vi "hex_ascii.vi"(11 "IN （HEX）":string) -> (3 "ASCII":string)   [LabVIEW 2015]
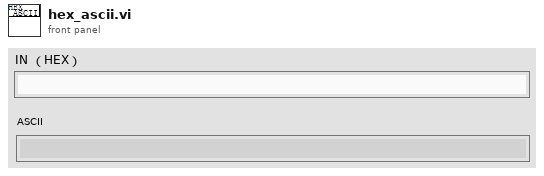
[diagram p1: front panel]
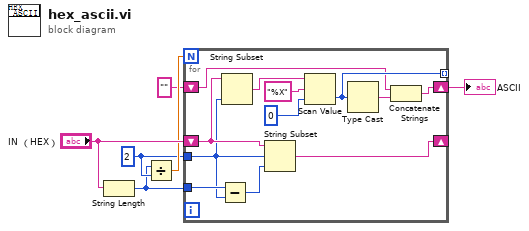
[diagram p0: block diagram]
diagram:
  w2 = 2 ("y")
  n1 = String Length(string="IN （HEX）") -> (length=w1:i32)
  n2 = Divide(x=w1, y=w2) -> (x/y=w5:dbl)
  n3 = for {
    N: w5 -> [_]
    shift-right: [w8] -> _
    shift-left: "IN （HEX）" -> [w12]
    tunnel: [w16] -> _ mode=indexing
    shift-right: [w13] -> w3
    shift-left: "" -> [w14]
    tunnel: w2 -> [w10]
    tunnel: w1 -> [w11]
    n4 = Subtract(x=w11, y=w10) -> (x-y=w9:i32)
    n5 = String Subset(string=w12, length (rest)=w10) -> (substring=w7:string)  [unwired: 1 in]
    n6 = String Subset(string=w12, offset (0)=w10, length (rest)=w9) -> (substring=w8:string)
    n7 = Scan Value(string=w7, format string="%X" ("格式字符串"), default (0 dbl)=i8 0 ("默认(0 dbl)")) -> (value=w16:i8)  [unwired: 1 out]
    n8 = Type Cast(x=w16) -> (*(type *) &x=w15:string)  [unwired: 1 in]
    n9 = Concatenate Strings(w14, w15) -> (w13:string)
  }
  "ASCII" <- w3
